vi "Test Data.vi"(0 "Size":i32=1) -> (1 "Data":variant, 2 "Timestamps":timestamp[](array[timestamp]))   [LabVIEW 2019]
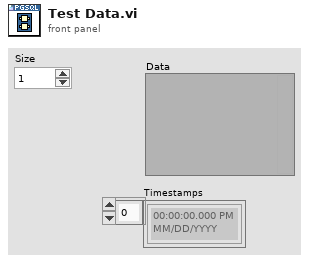
[diagram p1: front panel]
types:
  T1 = cluster{"integer":i32, "float":dbl, "string":string, "boolean":bool}
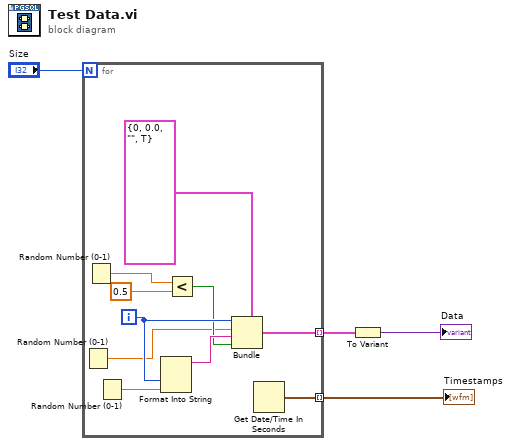
[diagram p0: block diagram]
diagram:
  n1 = for {
    N: "Size" -> [_]
    tunnel: [w8] -> w3 mode=indexing
    tunnel: [w5] -> w1 mode=indexing
    i -> [w14]
    n2 = Random Number (0-1)() -> (number: 0 to 1=w6:dbl)
    n3 = Random Number (0-1)() -> (number: 0 to 1=w12:dbl)
    n4 = Random Number (0-1)() -> (number: 0 to 1=w7:dbl)
    n5 = Format Into String(w14, w7) -> (resulting string=w13:string)  [unwired: 3 in, 1 out]
    n6 = Less?(x=w12, y=0.5) -> (x < y?=w10:bool)
    n7 = Bundle(cluster=T1 {"integer"=0, "float"=0.0, "string"="", "boolean"=TRUE}, "integer"=w14, "float"=w6, "string"=w13, "boolean"=w10) -> (w8:T1)
    n8 = Get Date/Time In Seconds() -> (seconds since 1Jan1904=w5:timestamp)
  }
  "Timestamps" <- w1
  n9 = To Variant(anything=w3) -> (Variant=→"Data":variant)
